vi "Park_from_EoL.vi"(3 "offset Y":dbl, 5 "offset X":dbl, 6 "Line_start":i32, 7 "Range":dbl=10.0, 8 "Pixels":i32=256, 9 "dwell":dbl=1.0) -> (0 "X and Y":waveform(dbl)[](array[waveform]), 1 "Array Y":dbl[](array[numeric]), 2 "Array X":dbl[](array[numeric]))   [LabVIEW 2016]
panel:
  out "start line Y":dbl
  out "Waveform Graph":waveform(dbl)[](graph)
  out "start line X":dbl
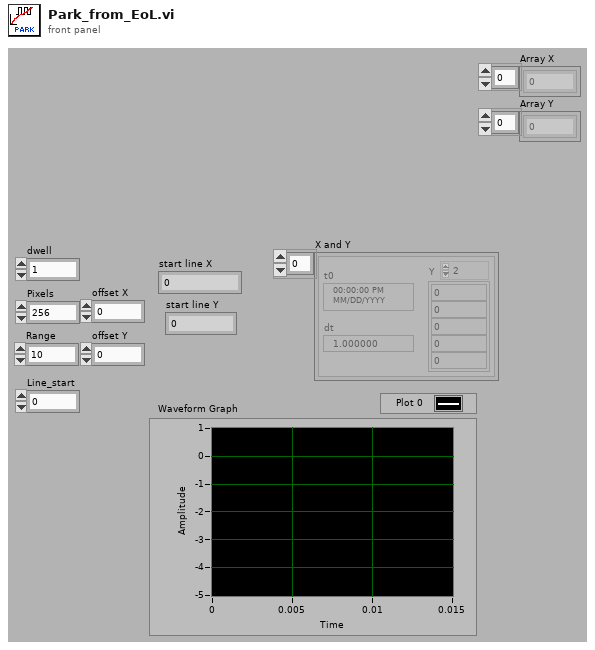
[diagram p1: front panel]
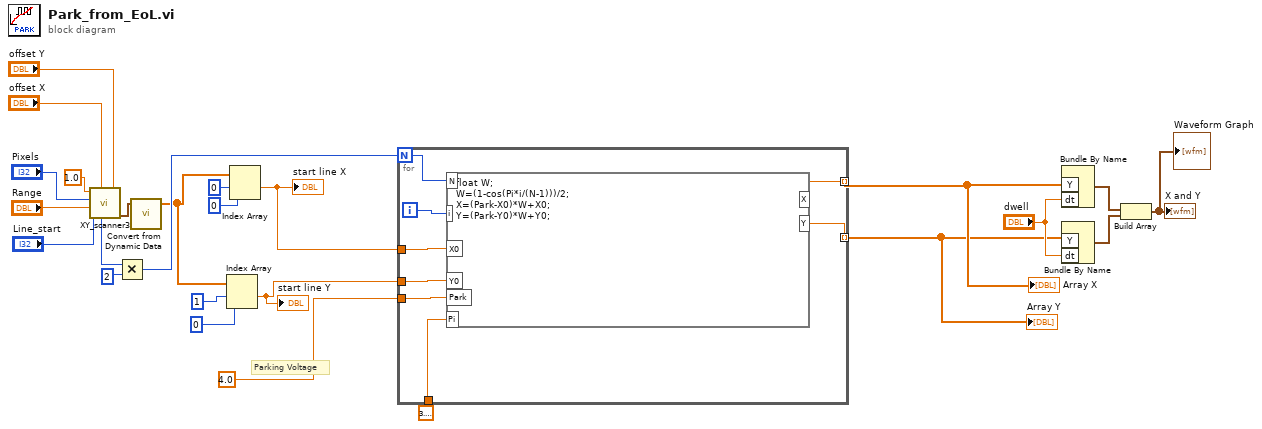
[diagram p0: block diagram]
diagram:
  # "Parking Voltage"
  n1 = call "XY_scanner3.vi"("offset Y"="offset Y", "offset X"="offset X", "Line_start"="Line_start", "Range"="Range", "Pixels"="Pixels", "dwell"=1.0) -> ("X and Y"=w1:waveform(dbl)[], "scanPix"=w15:i32)  [unwired: 2 out]
  n2 = Multiply(x=w15, y=2) -> (x*y=w14:i32)
  n3 = call "Convert from Dynamic Data"("Dynamic Data Type"=w1) -> ("Array"=w6:dbl[])  [unwired: 3 in]
  n4 = Index Array(array=w6, index #1=1 ("index"), index #2=0 ("index")) -> (element #1=w5:dbl)  [unwired: 1 out]
  "start line Y" <- w5
  n5 = Index Array(array=w6, index #1=0 ("index"), index #2=0 ("index")) -> (element #1=w9:dbl)  [unwired: 1 out]
  "start line X" <- w9
  n6 = for {
    N: w14 -> [w32]
    tunnel: 3.141592653589793 -> [w31]
    tunnel: [w30] -> w3 mode=indexing
    tunnel: [w29] -> w2 mode=indexing
    tunnel: w9 -> [w28]
    tunnel: w5 -> [w27]
    tunnel: 4.0 ("input variable") -> [w26]
    i -> [w33]
    n7 = formula code="float W;\nW=(1-cos(Pi*i/(N-1)))/2;\nX=(Park-X0)*W+X0;\nY=(Park-Y0)*W+Y0;"("N"=w32, "i"=w33, "Pi"=w31, "X0"=w28, "Y0"=w27, "Park"=w26) -> ("X"=w30:dbl, "Y"=w29:dbl)
  }
  "Array X" <- w3
  "Array Y" <- w2
  n8 = Bundle By Name("Y"=w3, "dt"="dwell") -> (w20:waveform(dbl))  [unwired: 1 in]
  n9 = Bundle By Name("Y"=w2, "dt"="dwell") -> (w19:waveform(dbl))  [unwired: 1 in]
  n10 = Build Array(w20, w19) -> (→"X and Y" →"Waveform Graph":waveform(dbl)[])
